vi "debouncer (SubVI).vi"(1 "Touch in Prev":bool, 2 "Touch in":bool) -> (0 "Touch out":bool)   [LabVIEW 2013]
doc: "Smooth touch input by filtering out a brief (single sample) lapse in touch.\n\nTruth table:\nTouch in | Touch in previous | Touch out\nTrue | True | True\nTrue | False | True\nFalse | True | True\nFalse | False | False"
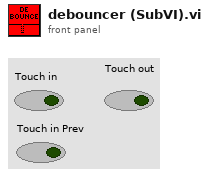
[diagram p1: front panel]
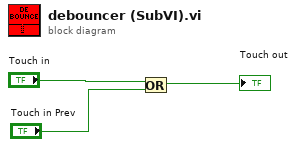
[diagram p0: block diagram]
diagram:
  n1 = Or(x="Touch in", y="Touch in Prev") -> (x .or. y?=→"Touch out":bool)
